vi "Write Primary Key.vi"(8 "error in (no error)":errorcluster, 10 "Primary Key":string, 11 "Table Configuration in":refnum<class "Table Configuration.lvclass">) -> (0 "error out":errorcluster, 3 "Table Configuration out":refnum<class "Table Configuration.lvclass">)   [LabVIEW 2020, in "Table.lvlib" / "Table Configuration.lvclass"]
uses:
  Table Configuration.lvclass
  Table Configuration.lvclass/Table Configuration.ctl
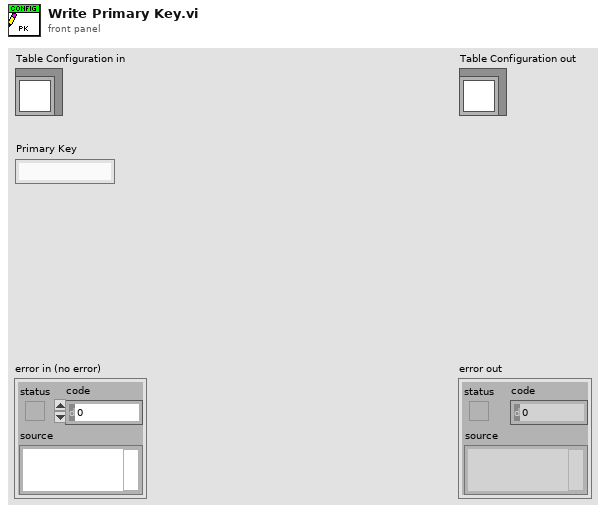
[diagram p1: front panel]
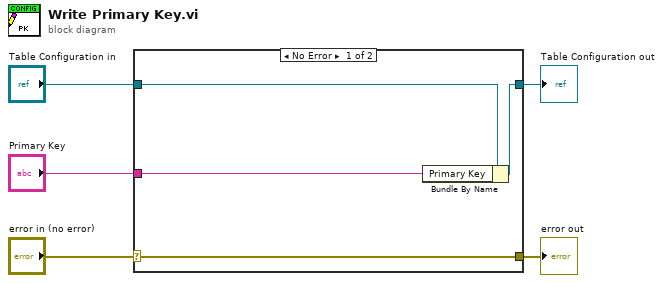
[diagram p0: block diagram]
diagram:
  n1 = case shown="No Error" "error in (no error)" {
    selector: "error in (no error)" -> [w9 w10]
    tunnel: [w9 w10] -> w4
    tunnel: [w7 w11] -> w2
    tunnel: "Table Configuration in" -> [w8 w11]
    tunnel: "Primary Key" -> [w6 _]
    frame No Error {
      n2 = Bundle By Name(cluster=w8, "Primary Key"=w6) -> (w7:refnum<class "Table Configuration.lvclass">)
    }
    frame Error {
    }
  }
  "error out" <- w4
  "Table Configuration out" <- w2
